vi "CalculateImageSize.vi"(8 "error in (no error)":errorcluster, 10 "String":string, 11 "Code128 in":refnum<class "Code128.lvclass">) -> (0 "error out":errorcluster, 2 "Size":cluster{"x":i16, "y":i16}, 3 "Code128 out":refnum<class "Code128.lvclass">)   [LabVIEW 2013, in "BarCodes.lvlib" / "Code128.lvclass"]
doc: "Calculates the size of the image for the barcode. This should include the entire barcode, quiet space, and text around it."
uses:
  Code128.lvclass
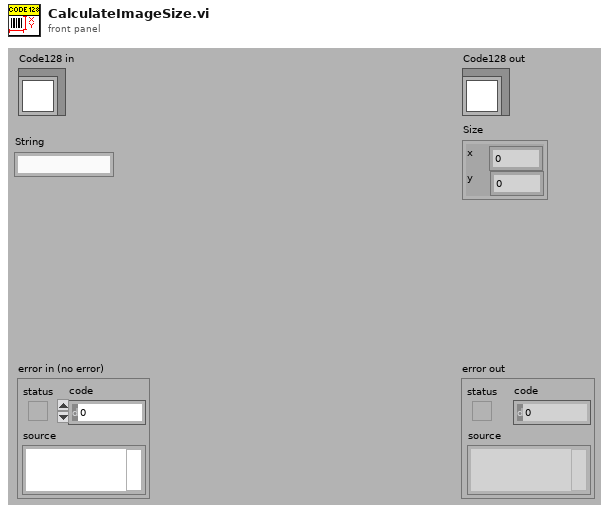
[diagram p1: front panel]
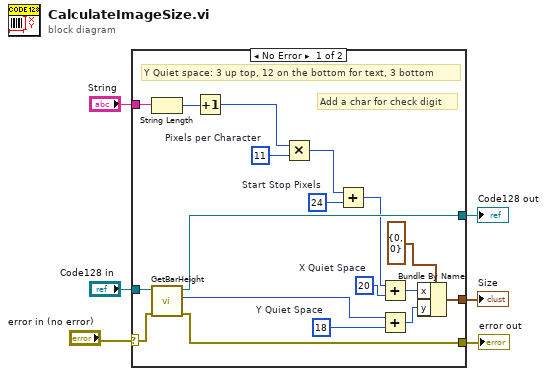
[diagram p0: block diagram]
diagram:
  n1 = case shown="No Error" "error in (no error)" {
    selector: "error in (no error)" -> [w8 w26]
    tunnel: "String" -> [w24 _]
    tunnel: "Code128 in" -> [w23 w25]
    tunnel: [w22 w26] -> w4
    tunnel: [w21 w25] -> w3
    tunnel: [w9 _] -> w2
    frame No Error {
      w13 = 20  # X Quiet Space
      w15 = 24  # Start Stop Pixels
      w17 = 11  # Pixels per Character
      w19 = u8 18  # Y Quiet Space
      # "Add a char for check digit"
      # "Y Quiet space: 3 up top, 12 on the bottom for text, 3 bottom"
      n2 = String Length(string=w24) -> (length=w18:i32)
      n3 = call-dynamic "GetBarHeight.vi"("error in (no error)"=w8, "Code128 in"=w23) -> ("error out"=w22:errorcluster, "Bar Height"=w20:u8, "Code128 out"=w21:refnum<class "Code128.lvclass">)  [unwired: 7 in]
      n4 = Increment(x=w18) -> (x+1=w7:i32)
      n5 = Multiply(x=w7, y=w17) -> (x*y=w16:i32)
      n6 = Add(x=w16, y=w15) -> (x+y=w14:i32)
      n7 = Add(x=w14, y=w13) -> (x+y=w11:i32)
      n8 = Add(x=w20, y=w19) -> (x+y=w10:u8)
      n9 = Bundle By Name(cluster=cluster{"x":i16, "y":i16} {"x"=0, "y"=0} ("Size"), "x"=w11, "y"=w10) -> (w9:cluster{"x":i16, "y":i16})
    }
    frame Error {
    }
  }
  "error out" <- w4
  "Code128 out" <- w3
  "Size" <- w2
